vi "Set Panes to Origins.vi"(8 "error in (no error)":errorcluster, 11 "Popup ViewManager In":refnum<class "Popup ViewManager.lvclass">) -> (0 "error out":errorcluster, 3 "Popup ViewManager Out":refnum<class "Popup ViewManager.lvclass">)   [LabVIEW 2017, in "Popup ViewManager.lvlib" / "Popup ViewManager.lvclass"]
doc: "<License>\nCopyright © 2017 Composed Systems, LLC | All rights reserved\nwww.composed.io\n\nAuthor: Ethan Stern <ethan.stern@composed.io>\n\nThis software is provided \"AS IS\" WITHOUT WARRANTIES, either express or implied, AND IS FOR EDUCATIONAL PURPOSES ONLY.\n</License>"
uses:
  <vilib>/gpm_packages/@cs/popup-viewmanager/Source/Popup ViewManager/Popup ViewManager.lvclass
  <vilib>/gpm_packages/@cs/popup-viewmanager/Source/Popup ViewManager/Popup ViewManager.lvclass/Popup ViewManager.ctl
  <vilib>/ActorFramework/Message Enqueuer/Message Enqueuer.lvclass/Message Enqueuer.ctl
  <vilib>/ActorFramework/Message Enqueuer/Enqueue.vi
  <vilib>/gpm_packages/@cs/mva-viewable/Source/IViewable/IViewable Messages/Set Panes to Origins Msg/Set Panes to Origins Msg.lvclass
  C:/Program Files/National Instruments/LabVIEW 2017/vi.lib/ActorFramework/Message/Message.lvclass
  <vilib>/ActorFramework/Message Priority Queue/Priority Enqueue.vi
  <vilib>/gpm_packages/@cs/mva-dialogbox/source/IDialogBox/IDialogBox/IDialogBox.lvclass
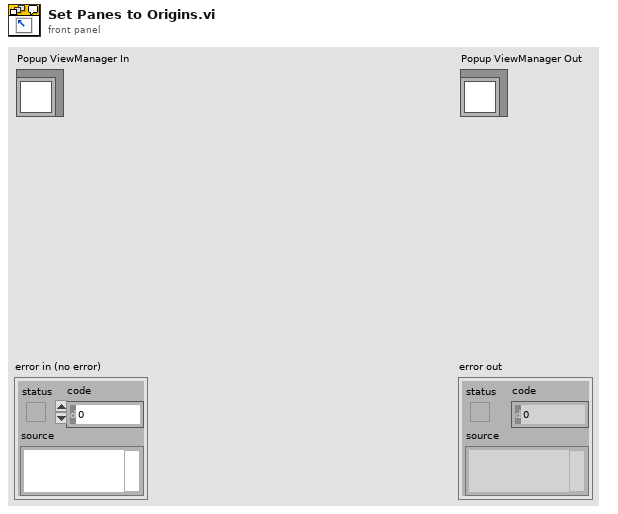
[diagram p1: front panel]
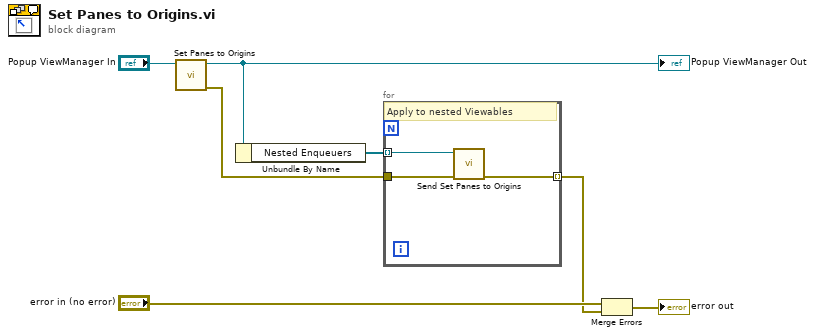
[diagram p0: block diagram]
diagram:
  n1 = call-parent "Set Panes to Origins.vi"("IViewable In"="Popup ViewManager In") -> ("error out"=w4:errorcluster, "IViewable Out"=w6:refnum<class "Popup ViewManager.lvclass">)  [unwired: 9 in]
  "Popup ViewManager Out" <- w6
  n2 = Unbundle By Name(w6) -> ("Nested Enqueuers"=w5:refnum<class "Message Enqueuer.lvclass">[])
  n3 = for {
    tunnel: w5 -> [w10] mode=indexing
    tunnel: w4 -> [w9]
    tunnel: [w8] -> w1 mode=indexing
    # "Apply to nested Viewables"
    n4 = call <vilib>:"Send Set Panes to Origins.vi"("error in (no error)"=w9, "Message Enqueuer"=w10) -> ("error out"=w8:errorcluster)  [unwired: 8 in, 1 out]
  }
  n5 = Merge Errors("error in (no error)", w1) -> (→"error out":errorcluster)
